vi "York DIHB - Data Processing - Oversampling and Interpolation.vi"() -> ()   [LabVIEW 2020]
uses:
  <vilib>/Utility/file.llb/Read Delimited Spreadsheet (DBL).vi
panel:
  out "First Peak":waveform(dbl)(graph)
  in  "Bits of Precision Increase":i32=1
  out "Interpolated Signal":waveform(dbl)(graph)
  out "Samples":i32
  out "Sampling Rate (MHz)":dbl
  out "Sampling Period (s)":dbl
  out "Raw Data - Strain Amplifier Output (Volts)":waveform(dbl)(graph)
  out "Projectile Velocity (m/s)":dbl
  out "Strain Amplifier (Volts)":dbl[](array[numeric])
  out "Time (Seconds)":dbl[](array[numeric])
  # "SET INTERPOLATION LEVEL, THE PRESS RUN TO SELECT THE DATA FILE"
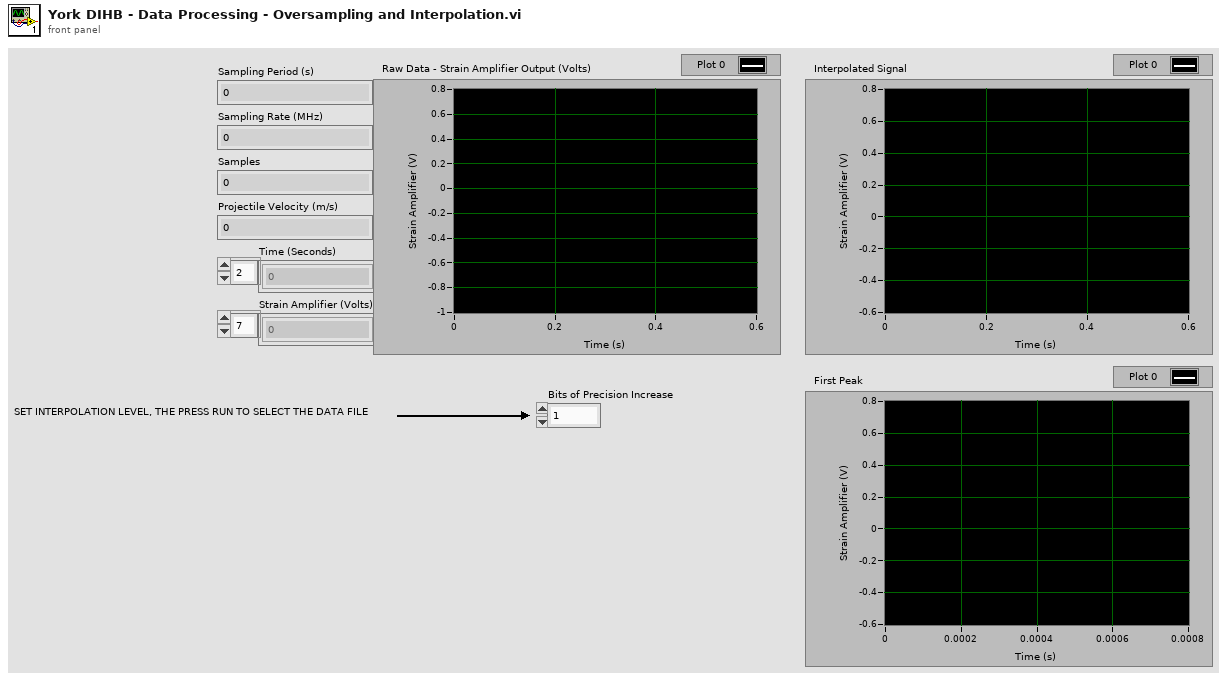
[diagram p1: front panel]
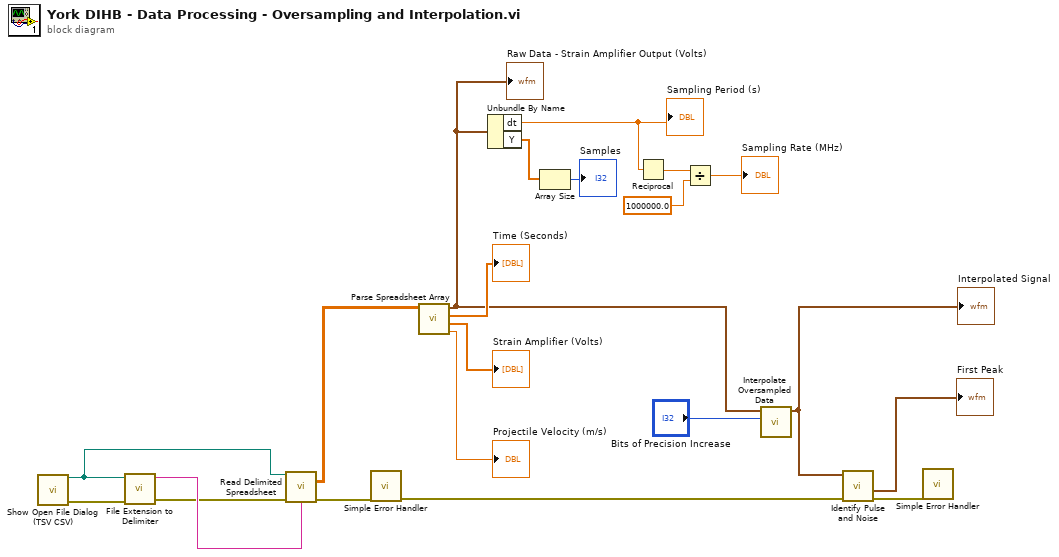
[diagram p0: block diagram]
diagram:
  n1 = call "Show Open File Dialog (TSV CSV).vi"() -> ("error out"=w7:errorcluster, "selected path"=w6:path)  [unwired: 10 in]
  n2 = call "File Extension to Delimiter.vi"("error in"=w7, "Data File Path"=w6) -> ("error out"=w5:errorcluster, "Delimiter"=w8:string)  [unwired: 8 in]
  n3 = call-poly <vilib>:"Read Delimited Spreadsheet.vi"("file path (dialog if empty)"=w6, "error in (no error)"=w5, "delimiter (\\t)"=w8) -> ("all rows"=w4:dbl[][], "error out"=w3:errorcluster)  [unwired: 7 in, 4 out]
  n4 = call <vilib>:"Simple Error Handler.vi"("error in (no error)"=w3) -> ("error out"=w2:errorcluster)  [unwired: 4 in, 4 out]
  n5 = call "Parse Spreadsheet Array.vi"("all rows"=w4) -> ("Projectile Velocity (m/s)"=→"Projectile Velocity (m/s)":dbl, "Strain Amplifier (Volts)"=→"Strain Amplifier (Volts)":dbl[], "Time (Seconds)"=→"Time (Seconds)":dbl[], "Waveform"=w11:waveform(dbl))  [unwired: 7 in]
  "Raw Data - Strain Amplifier Output (Volts)" <- w11
  n6 = Unbundle By Name(w11) -> ("dt"=w18:dbl, "Y"=w13:dbl[])
  "Sampling Period (s)" <- w18
  n7 = Array Size(array=w13) -> (size(s)=→"Samples":i32)
  n8 = Reciprocal(x=w18) -> (1/x=w17:dbl)
  n9 = Divide(x=w17, y=1000000.0) -> (x/y=→"Sampling Rate (MHz)":dbl)
  n10 = call "Interpolate Oversampled Data.vi"("Bits of Precision Increase"="Bits of Precision Increase", "Waveform in"=w11) -> ("Waveform out"=w10:waveform(dbl))  [unwired: 9 in]
  "Interpolated Signal" <- w10
  n11 = call "Identify Pulse and Noise.vi"("error in"=w2, "Waveform In"=w10) -> ("error out"=w1:errorcluster, "Signal Waveform Out"=→"First Peak":waveform(dbl))  [unwired: 5 in, 3 out]
  n12 = call <vilib>:"Simple Error Handler.vi"("error in (no error)"=w1) -> ()  [unwired: 4 in, 5 out]
